vi "002_DataSave.vi"(11 "Queue Ref":T1={"UI"=refnum, "Message"=refnum, "Data"=refnum, "Caller"=refnum, "Name"="000 Common", "Data Path"=path "", "Class Path"=path "", "SubPanel"=refnum, "Project Name"="", "MNT"="", "Title"="", "Data Source"=refnum, "Queue List"={}, "VI"=refnum, "UE"=refnum}) -> ()   [LabVIEW 2020]
doc: "DataSave"
uses:
  Alin/QMH/000 Module Data Type.ctl
  Alin/QMH/Queue Message.ctl
  <vilib>/Utility/config.llb/Read Key (String).vi
  <vilib>/Utility/config.llb/Write Key (String).vi
  <vilib>/Utility/config.llb/NI_LVConfig.lvlib
panel:
  in  "Data Save Edit":bool
  in  "Open Save Folder":bool
  in  "Data Save List":i32(listbox)
  in  "Data Graph Edit":bool
  in  "Open Graph Folder":bool
  in  "Data Graph List":i32(listbox)
  in  "Data Save Launch":bool
  in  "Data Save Interval":sgl=100.0 caption="存储间隔" min=0.1 max=3600 step=0.1 format="%#_g s"
  in  "Data Save Refresh":bool
  in  "Panel Show":bool
  in  "Save Info":i32(listbox) caption="操作日志"
  in  "Data Save Log":i32(listbox)
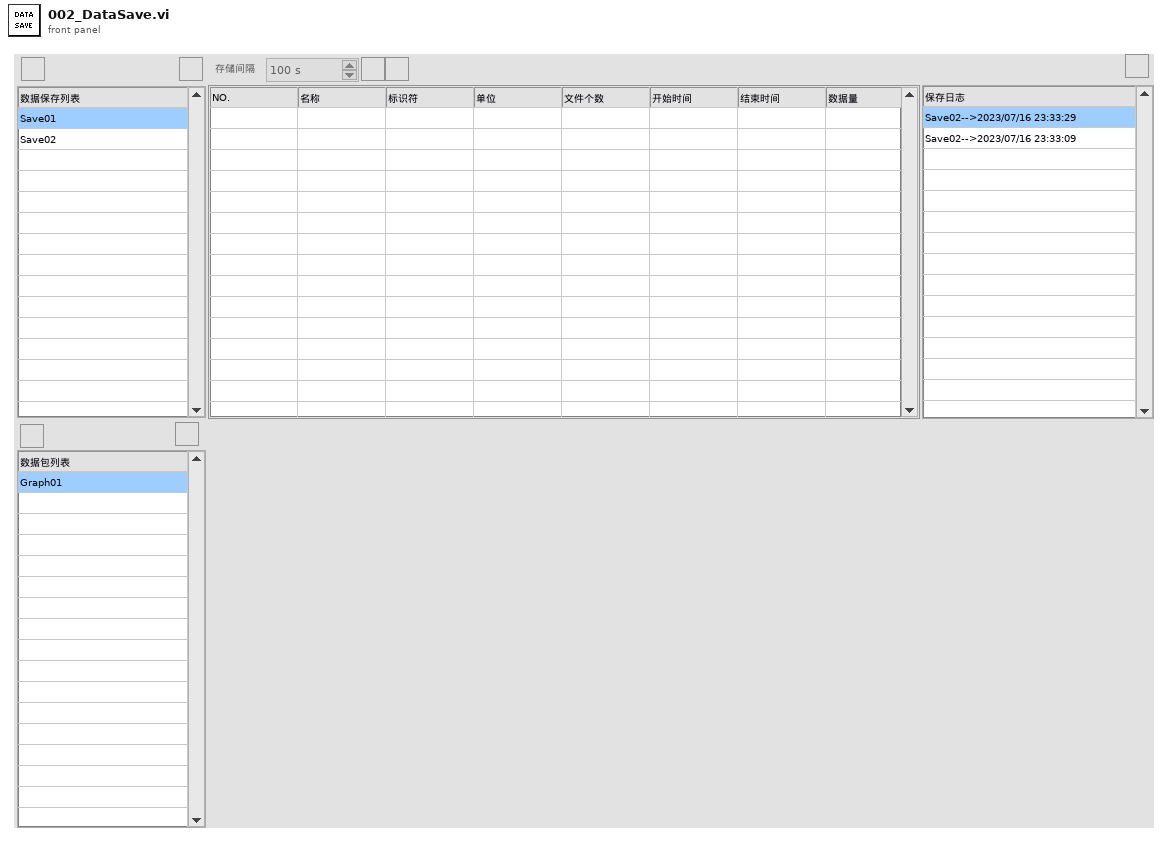
[diagram p1: front panel]
types:
  T1 = typedef "000 Module Data Type.ctl" = cluster{"UI":refnum<queue>, "Message":refnum<queue>, "Data":refnum<queue>, "Caller":refnum<queue>, "Name":string, "Data Path":path, "Class Path":path, "SubPanel":refnum<vi>, "Project Name":string, "MNT":string, "Title":string, "Data Source":refnum<queue>, "Queue List":map{string, refnum<queue>}, "VI":refnum<vi>, "UE":refnum<user-event>}
  T2 = cluster{"Queue":T1, "Data Save Log":refnum<vi>, "Log":string[]}
  T3 = typedef "eventvkey.ctl" = enum16{"ASCII", "Enter", "Return", "Shift", "Ctrl", "Alt", "Cmd", "Opt", "Caps", "NumLock", "Clear", "Break", "Up", "Down", "Left", "Right", "Insert", "Delete", "Home", "End", "PageUp", "PageDown", "Escape", "Help", "Pause", "ScrollLock", "F1", "F2", "F3", "F4", "F5", "F6", "F7", "F8", "F9", "F10", "F11", "F12", "F13", "F14", "F15", "F16", "F17", "F18", "F19", "F20", "F21", "F22", "F23", "F24", "Play", "VolumeUp", "VolumeDown", "Mute", "Two Byte Char"}
  T4 = cluster{"Shift":bool, "Ctrl":bool, "Alt":bool, "Cmd":bool, "Opt":bool}
  T5 = cluster{"Queue List":map{string, refnum<queue>}, "SubPanel":refnum<vi>, "Queue":T1, "Graph List":refnum<vi>, "Save List":refnum<vi>, "Save Info":refnum<vi>, "Active Save":string, "SQ":map{string, refnum<user-event>}}
  T6 = enum8{"Enabled", "Disabled", "Disabled and Grayed Out"}
  T7 = typedef "NI_LVConfig.lvlib/Config Data RefNum.ctl" = refnum<k1>
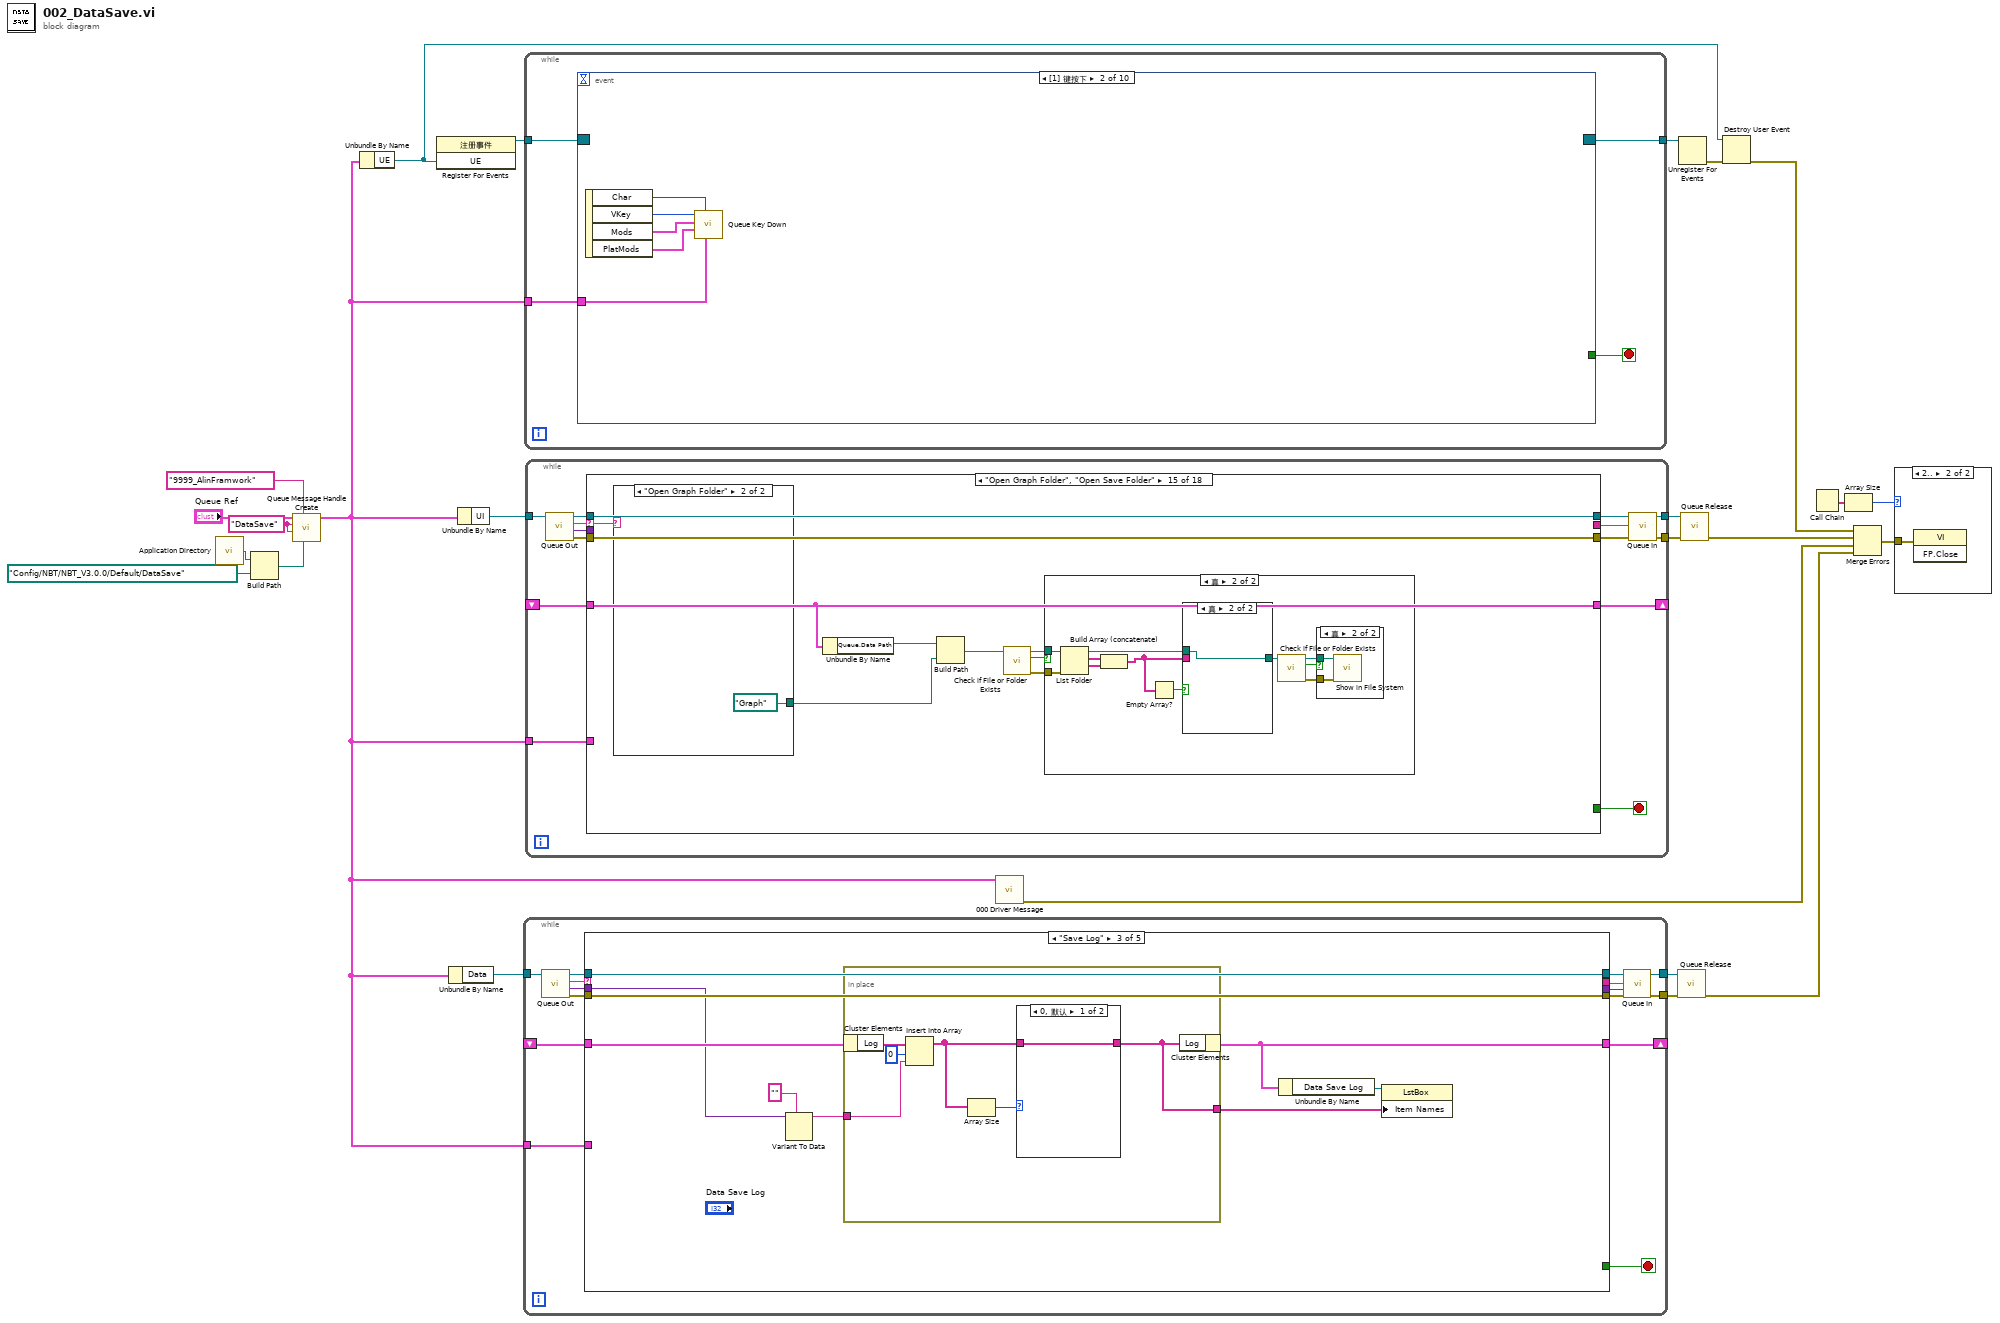
[diagram p0: block diagram]
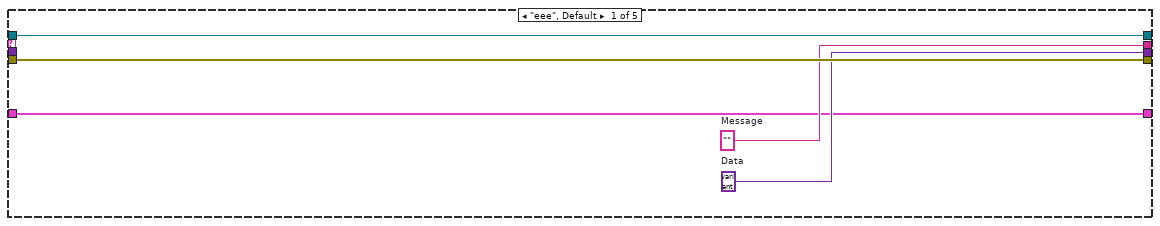
[diagram p2: hidden frame]
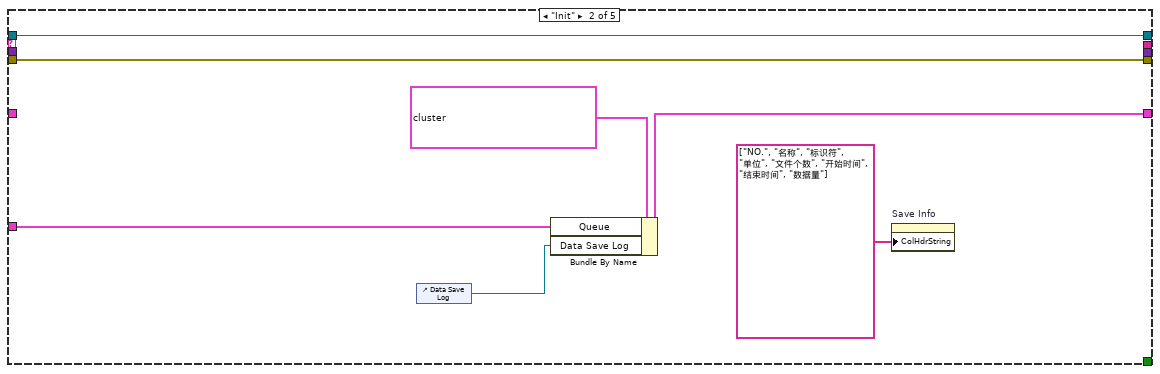
[diagram p3: hidden frame]
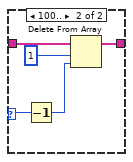
[diagram p4: hidden frame]
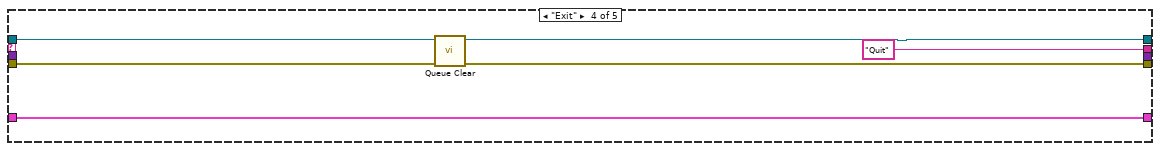
[diagram p5: hidden frame]
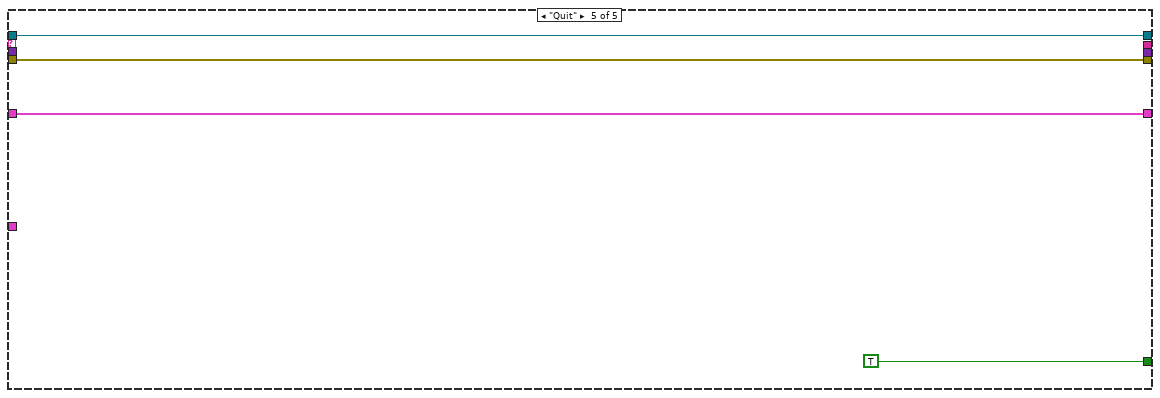
[diagram p6: hidden frame]
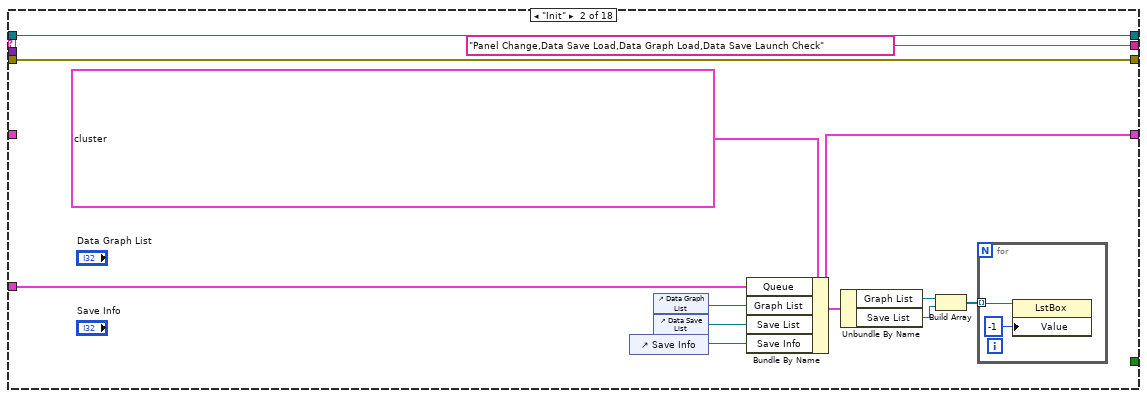
[diagram p9: hidden frame]
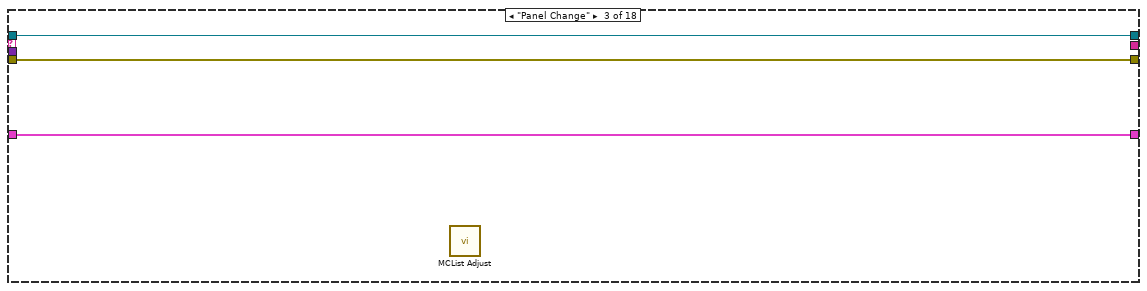
[diagram p10: hidden frame]
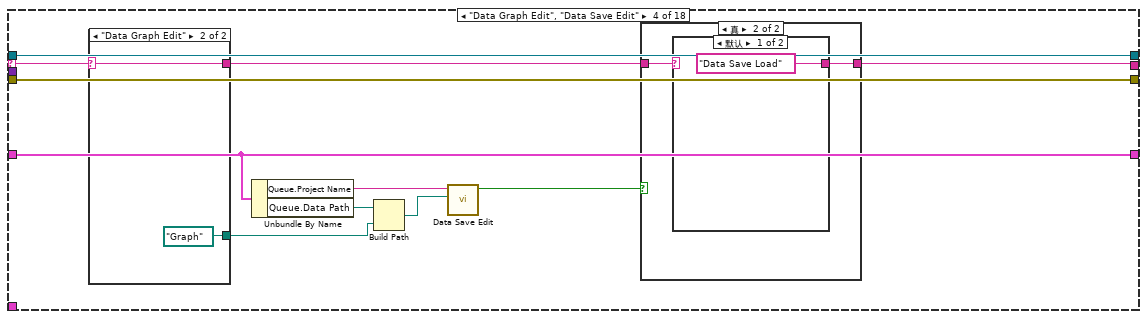
[diagram p11: hidden frame]
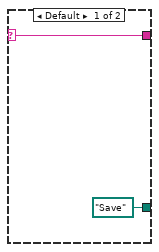
[diagram p12: hidden frame]
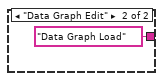
[diagram p14: hidden frame]
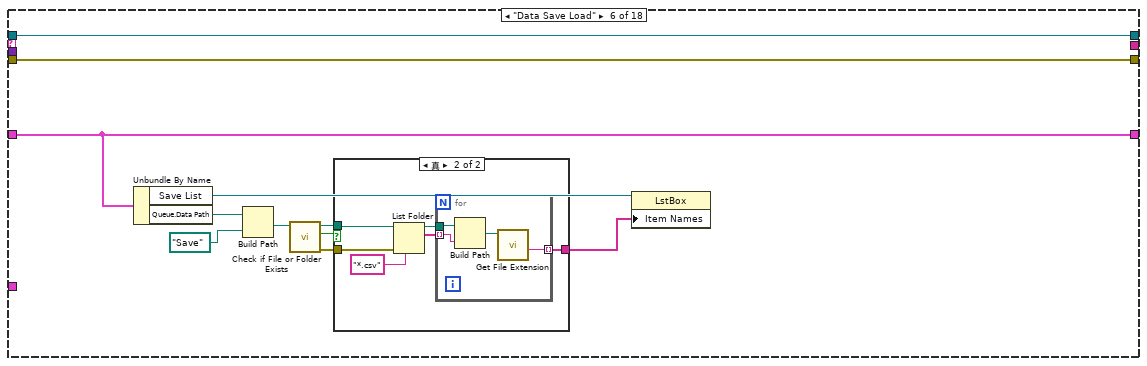
[diagram p16: hidden frame]
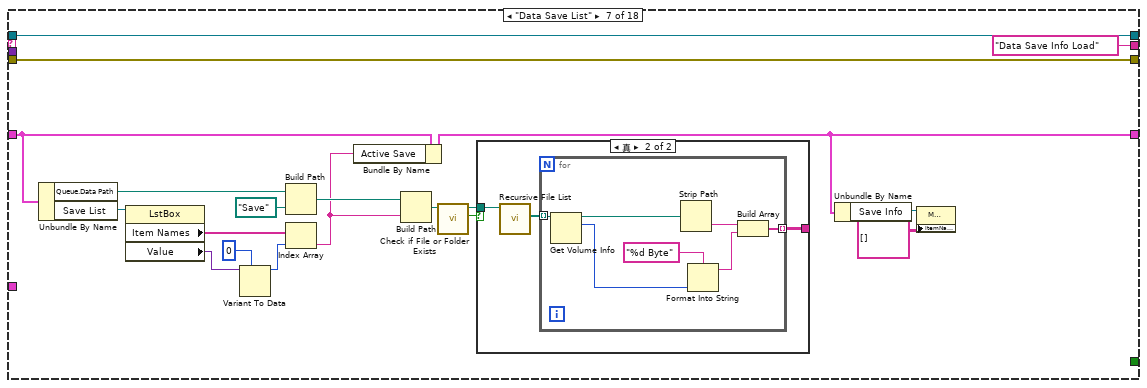
[diagram p18: hidden frame]
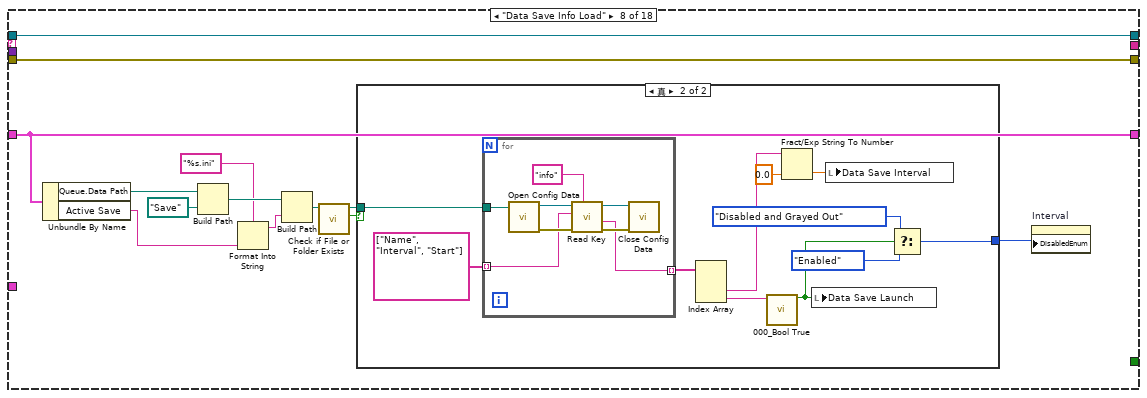
[diagram p20: hidden frame]
diagram:
  w2 = "DataSave" ("Title")
  n1 = call <vilib>:"Application Directory.vi"() -> ("Application Directory"=w5:path)
  n2 = Build Path(base path=w5, name or relative path=path "Config/NBT/NBT_V3.0.0/Default/DataSave" ("名称或相对路径")) -> (appended path=w3:path)
  n3 = call "Queue Message Handle Create.vi"("Data Path"=w3, "Project Name"="9999_AlinFramwork", "Name"=w2, "Title"=w2, "Queue Ref In"="Queue Ref") -> ("Queue Ref Out"=w7:T1)  [unwired: 5 in, 1 out]
  n4 = Unbundle By Name(w7) -> ("UE"=w6:refnum<user-event>)
  n5 = register-events(w6) -> (reference out=w9:refnum<event-registration>)  [unwired: 2 in, 1 out]
  n6 = Unbundle By Name(w7) -> ("Data"=w22:refnum<queue>)
  n7 = Unbundle By Name(w7) -> ("UI"=w14:refnum<queue>)
  n8 = while {
    tunnel: w22 -> [w35]
    tunnel: [w32] -> w20
    tunnel: [w31] -> w21
    shift-right: [w27] -> _
    shift-left: _ -> [w26]
    tunnel: w7 -> [w25]
    stop <- w39 stop-if-true
    n9 = call "Queue Out.vi"("Queue In"=w35) -> ("error out"=w38:errorcluster, "Data"=w36:variant, "Message"=w37:string, "Queue Out"=w34:refnum<queue>)  [unwired: 6 in, 1 out]
    n10 = case shown="\"Save Log\"" w37 {
      tunnel: w34 -> [w44 w51 w60 w77 w81]
      tunnel: w38 -> [w43 w50 w59 w75 w82]
      tunnel: [w44 w51 w60 w76 w81] -> w33
      tunnel: [w43 w50 w59 w74 w82] -> w30
      tunnel: [w42 _ _ "Quit" _] -> w29
      tunnel: [_ _ _ _ TRUE] -> w39
      tunnel: [w41 _ _ _ _] -> w28
      tunnel: w36 -> [_ _ w57 _ _]
      tunnel: [w40 w47 w54 w73 w79] -> w27
      tunnel: w26 -> [w40 _ w58 w73 w79]
      tunnel: w25 -> [_ w48 _ _ _]
      frame "eee", Default {
        w41 = variant  # Data
        w42 = ""  # Message
      }
      frame "Init" {
        n11 = control-ref of="Data Save Log"() -> (w45:refnum<vi>)
        n12 = Bundle By Name(cluster=T2 {"Queue"={"UI"=refnum, "Message"=refnum, "Data"=refnum, "Caller"=refnum, "Name"="", "Data Path"=path "", "Class Path"=path "", "SubPanel"=refnum, "Project Name"="", "MNT"="", "Title"="", "Data Source"=refnum, "Queue List"={}, "VI"=refnum, "UE"=refnum}, "Data Save Log"=refnum, "Log"=[]}, "Queue"=w48, "Data Save Log"=w45) -> (w47:T2)
        n13 = property on="Save Info" class="MCListbox (严格)"("ColHdrString"=string[] ["NO.", "名称", "标识符", "单位", "文件个数", "开始时间", "结束时间", "数据量"] ("列首字符串[]")) -> ()  [unwired: 2 in, 2 out]
      }
      frame "Save Log" {
        n14 = Variant To Data(type="", Variant=w57) -> (data=w55:string)  [unwired: 1 in, 1 out]
        n15 = in-place {
          in-place-border: w55 -> [w65]
          in-place-border: [w61] -> w52
          n16 = in-place-cluster #1(w58) -> ("Log"=w66:string[])
          n17 = Insert Into Array(array=w66, index=0 ("索引"), new element=w65) -> (w63:string[])
          n18 = Array Size(array=w63) -> (size(s)=w62:i32)
          n19 = case shown="0, 默认" w62 {
            selector: w62 -> [_ w69]
            tunnel: w63 -> [w67 w72]
            tunnel: [w67 w71] -> w61
            frame 0, Default {
            }
            frame 100.. {
              n20 = Decrement(x=w69) -> (x-1=w68:i32)
              n21 = Delete From Array(array=w72, length=1 ("长度"), index=w68) -> (array with subset deleted=w71:string[])  [unwired: 1 out]
            }
          }
          n22 = in-place-cluster #1("Log"=w61) -> (w54:T2)
        }
        n23 = Unbundle By Name(w54) -> ("Data Save Log"=w53:refnum<vi>)
        n24 = property class="LstBox"(reference=w53, "Item Names"=w52) -> ()  [unwired: 1 in, 2 out]
      }
      frame "Exit" {
        n25 = call "Queue Clear.vi"("error in (no error)"=w75, "Queue In"=w77) -> ("error out"=w74:errorcluster, "Queue Out"=w76:refnum<queue>)  [unwired: 8 in]
      }
      frame "Quit" {
      }
    }
    n26 = call "Queue In.vi"("error in (no error)"=w30, "Data"=w28, "Message"=w29, "Queue In"=w33) -> ("error out"=w31:errorcluster, "Queue Out"=w32:refnum<queue>)  [unwired: 6 in]
  }
  n27 = while {
    tunnel: w9 -> [w86]
    tunnel: [w84] -> w10
    tunnel: w7 -> [w83]
    stop <- w85 stop-if-true
    n28 = event shown="[1] 键按下" {
      selector: w86 -> [_ _ _ _ _ _ _ _ _ _]
      dyn-events: [_ _ _ _ _ _ _ _ _ _] -> w84
      timeout: _ -> [_ _ _ _ _ _ _ _ _ _]
      tunnel: [_ _ _ _ _ w103 _ _ _ _] -> w85
      tunnel: w83 -> [_ w90 w95 w99 w102 _ w107 w117 w120 w124]
      event Timeout {
        n29 = event-data() -> ()  [unwired: 1 in, 1 out]
      }
      event Key Down {
        n30 = event-data() -> ("Char"=w91:i16, "VKey"=w89:T3, "Mods"=w88:cluster{"Num Pad":bool, "Menu Key":bool}, "PlatMods"=w87:T4)  [unwired: 1 in]
        n31 = call "Queue Key Down.vi"("Queue Ref Out"=w90, "C"=w91, "Platform Key"=w87, "Group Key"=w88, "V Key"=w89) -> ()  [unwired: 6 in, 1 out]
      }
      event "Data Save Edit", "Data Graph Edit", "Data Save Launch", "Data Save Refresh": Value Change {
        n32 = event-data() -> ("CtlRef"=w94:refnum<vi>)  [unwired: 1 in]
        n33 = Unbundle By Name(w95) -> ("UI"=w93:refnum<queue>)
        n34 = property class="Bool"(reference=w94) -> ("Label.Text"=w92:string)  [unwired: 1 in, 2 out]
        n35 = call "Queue In.vi"("Message"=w92, "Queue In"=w93) -> ()  [unwired: 8 in, 2 out]
      }
      event "Data Save Interval": Value Change {
        n36 = event-data() -> ("CtlRef"=w97:refnum<vi>)  [unwired: 1 in]
        n37 = Unbundle By Name(w99) -> ("UI"=w98:refnum<queue>)
        n38 = property class="DigNum (严格)"(reference=w97) -> ("Label.Text"=w96:string)  [unwired: 1 in, 2 out]
        n39 = call "Queue In.vi"("Message"=w96, "Queue In"=w98) -> ()  [unwired: 8 in, 2 out]
      }
      event Panel Resize {
        n40 = event-data() -> ()  [unwired: 1 in, 1 out]
        n41 = Unbundle By Name(w102) -> ("Message"=w101:refnum<queue>)
        n42 = call "Queue In.vi"("Message"="Panel Change", "Queue In"=w101) -> ()  [unwired: 8 in, 2 out]
      }
      event User Event {
        n43 = event-data() -> ("Message"=w105:string)  [unwired: 1 in]
        n44 = Equal?(x=w105, y="Exit") -> (x = y?=w103:bool)
      }
      event Panel Close? {
        n45 = event-data() -> ()  [unwired: 1 in, 1 out]
        n46 = Unbundle By Name(w107) -> ("Message"=w106:refnum<queue>)
        n47 = Call Chain() -> (call chain=w110:string[])
        n48 = Array Size(array=w110) -> (size(s)=w109:i32)
        n49 = case shown="0, 默认" w109 {
          tunnel: ["Exit Prepare" ("Message") "Panel Hidden" ("Message")] -> w108
          frame 0, Default {
          }
          frame 2.. {
          }
        }
        n50 = call "Queue In.vi"("Message"=w108, "Queue In"=w106) -> ()  [unwired: 8 in, 2 out]
        n51 = event-data("Discard?"=TRUE ("放弃？")) -> ()  [unwired: 1 in, 1 out]
      }
      event "Data Save List", "Data Graph List", "Open Save Folder", "Open Graph Folder": Value Change {
        n52 = event-data() -> ("CtlRef"=w116:refnum<vi>)  [unwired: 1 in, 2 out]
        n53 = Unbundle By Name(w117) -> ("UI"=w115:refnum<queue>)
        n54 = property class="Ctl"(reference=w116) -> ("Label.Text"=w114:string)  [unwired: 1 in, 2 out]
        n55 = call "Queue In.vi"("Message"=w114, "Queue In"=w115) -> ()  [unwired: 8 in, 2 out]
      }
      event "Data Save List": Double Click {
        n56 = event-data() -> ()  [unwired: 1 in, 1 out]
        n57 = Unbundle By Name(w120) -> ("UI"=w119:refnum<queue>)
        n58 = call "Queue In.vi"("Message"="Show Panel", "Queue In"=w119) -> ()  [unwired: 8 in, 2 out]
      }
      event "Panel Show": Value Change {
        n59 = event-data() -> ("CtlRef"=w122:refnum<vi>)  [unwired: 1 in]
        n60 = Unbundle By Name(w124) -> ("Message"=w123:refnum<queue>)
        n61 = property class="Bool"(reference=w122) -> ("Label.Text"=w121:string)  [unwired: 1 in, 2 out]
        n62 = call "Queue In.vi"("Message"=w121, "Queue In"=w123) -> ()  [unwired: 8 in, 2 out]
      }
    }
  }
  n63 = while {
    tunnel: w14 -> [w134]
    tunnel: [w131] -> w12
    tunnel: [w130] -> w13
    tunnel: w7 -> [w127]
    shift-right: [w126] -> _
    shift-left: _ -> [w125]
    stop <- w138 stop-if-true
    n64 = call "Queue Out.vi"("Queue In"=w134) -> ("error out"=w137:errorcluster, "Data"=w135:variant, "Message"=w136:string, "Queue Out"=w133:refnum<queue>)  [unwired: 6 in, 1 out]
    n65 = case shown="\"Open Graph Folder\", \"Open Save Folder\"" w136 {
      selector: w136 -> [_ _ _ w161 _ _ _ _ _ _ _ _ _ w415 w425 _ w457 _]
      tunnel: w133 -> [w141 w153 w158 w169 w180 w191 w220 w243 w269 w282 w316 w343 w404 w421 w433 w456 w467 w477]
      tunnel: w137 -> [w140 w152 w157 w168 w179 w190 w219 w242 w268 w281 w315 w342 w403 w420 w432 w455 w465 w478]
      tunnel: [w141 w153 w158 w169 w180 w191 w220 w243 w269 w282 w316 w343 w404 w421 w433 w456 w466 w477] -> w132
      tunnel: [w140 w152 w157 w168 w179 w190 w219 w242 w268 w281 w315 w342 w403 w420 w432 w455 w464 w478] -> w129
      tunnel: [_ "Panel Change,Data Save Load,Data Graph Load,Data Save Launch Check" _ w162 _ _ "Data Save Info Load" _ w265 _ "Data Save Info Load,Data Save Launch Check" _ _ _ _ _ "Quit" _] -> w128
      tunnel: [_ _ _ _ _ _ _ _ _ _ _ _ _ _ _ _ _ TRUE] -> w138
      tunnel: w135 -> [_ _ _ _ _ _ _ _ _ _ _ _ _ _ _ _ _ _]
      tunnel: w127 -> [_ w150 _ _ _ _ _ _ _ _ _ _ _ _ _ _ _ _]
      tunnel: [w139 w145 w156 w167 w178 w189 w203 w237 w264 w279 w307 w340 w402 w419 w431 w454 w459 w475] -> w126
      tunnel: w125 -> [w139 _ w156 w167 w178 w189 w207 w237 w264 w280 w307 w331 w402 w419 w431 w454 w459 w475]
      frame "eee", Default {
      }
      frame "Init" {
        n66 = control-ref of="Save Info"() -> (w146:refnum<vi>)
        n67 = control-ref of="Data Graph List"() -> (w148:refnum<vi>)
        n68 = control-ref of="Data Save List"() -> (w147:refnum<vi>)
        n69 = Bundle By Name(cluster=T5 {"Queue List"={}, "SubPanel"=refnum, "Queue"={"UI"=refnum, "Message"=refnum, "Data"=refnum, "Caller"=refnum, "Name"="", "Data Path"=path "", "Class Path"=path "", "SubPanel"=refnum, "Project Name"="", "MNT"="", "Title"="", "Data Source"=refnum, "Queue List"={}, "VI"=refnum, "UE"=refnum}, "Graph List"=refnum, "Save List"=refnum, "Save Info"=refnum, "Active Save"="", "SQ"={}}, "Queue"=w150, "Graph List"=w148, "Save List"=w147, "Save Info"=w146) -> (w145:T5)
        n70 = Unbundle By Name(w145) -> ("Graph List"=w144:refnum<vi>, "Save List"=w143:refnum<vi>)
        n71 = Build Array(w144, w143) -> (w142:refnum<vi>[])
        n72 = for {
          tunnel: w142 -> [w155] mode=indexing
          n73 = property class="LstBox"(reference=w155, "Value"=-1) -> ()  [unwired: 1 in, 2 out]
        }
      }
      frame "Panel Change" {
        n74 = call "MCList Adjust.vi"() -> ()  [unwired: 11 in, 1 out]
      }
      frame "Data Graph Edit", "Data Save Edit" {
        n75 = case shown="\"Data Graph Edit\"" w161 {
          selector: w161 -> [w170 w172]
          tunnel: [path "Save" ("名称或相对路径") path "Graph" ("名称或相对路径")] -> w160
          tunnel: [w170 w172] -> w159
          frame Default {
          }
          frame "Data Graph Edit" {
          }
        }
        n76 = Unbundle By Name(w167) -> ("Queue.Project Name"=w166:string, "Queue.Data Path"=w164:path)
        n77 = Build Path(base path=w164, name or relative path=w160) -> (appended path=w163:path)
        n78 = call "Data Save Edit.vi"("Data Path"=w163, "Project"=w166) -> ("OK?"=w165:bool)  [unwired: 9 in]
        n79 = case shown="真" w165 {
          tunnel: [_ w175] -> w162
          tunnel: w159 -> [_ w174]
          frame False {
          }
          frame True {
            n80 = case shown="默认" w174 {
              tunnel: ["Data Save Load" "Data Graph Load"] -> w175
              frame Default {
              }
              frame "Data Graph Edit" {
              }
            }
          }
        }
      }
      frame "Data Save Delete" {
      }
      frame "Data Save Load" {
        n81 = Unbundle By Name(w189) -> ("Save List"=w182:refnum<vi>, "Queue.Data Path"=w188:path)
        n82 = Build Path(base path=w188, name or relative path=path "Save" ("名称或相对路径")) -> (appended path=w186:path)
        n83 = call <vilib>:"Check if File or Folder Exists.vi"("path"=w186) -> ("error out"=w183:errorcluster, "file or folder exists?"=w185:bool, "dup path"=w184:path)  [unwired: 8 in]
        n84 = case shown="真" w185 {
          tunnel: w184 -> [_ w197]
          tunnel: w183 -> [_ w196]
          tunnel: [_ w193] -> w181
          frame False {
          }
          frame True {
            n85 = List Folder(path=w197, pattern="*.csv" ("类型"), error in=w196) -> (path out=w194:path, filenames=w195:string[])  [unwired: 1 in, 2 out]
            n86 = for {
              tunnel: w195 -> [w200] mode=indexing
              tunnel: w194 -> [w201]
              tunnel: [w198] -> w193 mode=indexing
              n87 = Build Path(base path=w201, name or relative path=w200) -> (appended path=w199:path)
              n88 = call <vilib>:"Get File Extension.vi"("file"=w199) -> ("filename without extension"=w198:string)  [unwired: 6 in, 4 out]
            }
          }
        }
        n89 = property class="LstBox"(reference=w182, "Item Names"=w181) -> ()  [unwired: 1 in, 2 out]
      }
      frame "Data Save List" {
        n90 = Unbundle By Name(w207) -> ("Queue.Data Path"=w213:path, "Save List"=w218:refnum<vi>)
        n91 = property class="LstBox"(reference=w218) -> ("Item Names"=w217:string[], "Value"=w216:variant)  [unwired: 1 in, 2 out]
        n92 = Variant To Data(type=0 ("Data Save List"), Variant=w216) -> (data=w214:i32)  [unwired: 1 in, 1 out]
        n93 = Build Path(base path=w213, name or relative path=path "Save" ("名称或相对路径")) -> (appended path=w211:path)
        n94 = Index Array(array=w217, index=w214) -> (element=w202:string)
        n95 = Bundle By Name(cluster=w207, "Active Save"=w202) -> (w203:T5)
        n96 = Build Path(base path=w211, name or relative path=w202) -> (appended path=w210:path)
        n97 = call <vilib>:"Check if File or Folder Exists.vi"("path"=w210) -> ("file or folder exists?"=w209:bool, "dup path"=w208:path)  [unwired: 8 in, 1 out]
        n98 = case shown="真" w209 {
          tunnel: w208 -> [_ w223]
          tunnel: [_ w221] -> _
          frame False {
          }
          frame True {
            n99 = call <vilib>:"Recursive File List.vi"("Folder Path"=w223) -> ("All Files in Dir"=w222:path[])  [unwired: 6 in, 4 out]
            n100 = for {
              tunnel: w222 -> [w230] mode=indexing
              tunnel: [w224] -> w221 mode=indexing
              n101 = Get Volume Info(11:w230) -> (2:w227:i64, 3:w229:path)  [unwired: 1 in, 4 out]
              n102 = Strip Path(path=w229) -> (name=w226:string)  [unwired: 1 out]
              n103 = Format Into String(format string="%d Byte" ("格式字符串"), w227) -> (resulting string=w225:string)  [unwired: 2 in, 1 out]
              n104 = Build Array(w226, w225) -> (w224:string[])
            }
          }
        }
        n105 = Unbundle By Name(w203) -> ("Save Info"=w206:refnum<vi>)
        n106 = property class="MCListbox"(reference=w206, "ItemNames"=string[][] [] ("项名")) -> ()  [unwired: 1 in, 2 out]
      }
      frame "Data Save Info Load" {
        n107 = Unbundle By Name(w237) -> ("Queue.Data Path"=w241:path, "Active Save"=w232:string)
        n108 = Build Path(base path=w241, name or relative path=path "Save" ("名称或相对路径")) -> (appended path=w239:path)
        n109 = Format Into String(format string="%s.ini" ("格式字符串"), w232) -> (resulting string=w235:string)  [unwired: 2 in, 1 out]
        n110 = Build Path(base path=w239, name or relative path=w235) -> (appended path=w238:path)
        n111 = call <vilib>:"Check if File or Folder Exists.vi"("path"=w238) -> ("file or folder exists?"=w233:bool, "dup path"=w234:path)  [unwired: 8 in, 1 out]
        n112 = case shown="真" w233 {
          tunnel: w234 -> [_ w255]
          tunnel: [T6."Enabled" ("禁用") w245] -> w231
          frame False {
          }
          frame True {
            n113 = for {
              tunnel: w255 -> [w263]
              tunnel: string[] ["Name", "Interval", "Start"] -> [w257] mode=indexing
              tunnel: [w256] -> w253 mode=indexing
              n114 = call <vilib>:"Open Config Data.vi"("configuration file path"=w263) -> ("error out"=w261:errorcluster, "refnum"=w262:T7)  [unwired: 8 in, 1 out]
              n115 = call-poly <vilib>:"Read Key.vi"("section"="info", "error in (no error)"=w261, "key"=w257, "refnum"=w262) -> ("error out"=w260:errorcluster, "value"=w256:string, "refnum out"=w259:T7)  [unwired: 4 in, 1 out]
              n116 = call <vilib>:"Close Config Data.vi"("error in (no error)"=w260, "refnum"=w259) -> ()  [unwired: 8 in, 2 out]
            }
            n117 = Index Array(array=w253) -> (element #2=w252:string, element #3=w251:string)  [unwired: 3 in, 1 out]
            n118 = call "000_Bool True.vi"("Bool String"=w251) -> ("True"=w248:bool)  [unwired: 8 in, 2 out]
            n119 = Fract/Exp String To Number(string=w252, default (0 dbl)=sgl 0.0 ("偏移量")) -> (number=w250:sgl)  [unwired: 2 in, 1 out]
            n120 = local write "Data Save Launch"(w248) -> ()
            n121 = local write "Data Save Interval"(w250) -> ()
            n122 = Select(t=T6."Disabled and Grayed Out" ("禁用"), s=w248, f=T6."Enabled" ("禁用")) -> (s? t:f=w245:T6)
          }
        }
        n123 = property on="Interval" class="DigNum (严格)"("DisabledEnum"=w231) -> ()  [unwired: 2 in, 2 out]
      }
      frame "Data Save Launch" {
        n124 = local read "Data Save Launch"() -> (w267:bool)
        n125 = case shown="真" w267 {
          tunnel: [_ w277] -> w266
          tunnel: w264 -> [_ w276]
          frame False {
          }
          frame True {
            n126 = local read "Data Save Interval"() -> (w273:sgl)
            n127 = Unbundle By Name(w276) -> ("Active Save"=w274:string)
            n128 = Format Into String(format string="保存名称：%s\n保存间隔：%#.3f s" ("格式字符串"), w274, w273) -> (resulting string=w272:string)  [unwired: 2 in, 1 out]
            n129 = Two Button Dialog(message=w272) -> (T button?=w277:bool)  [unwired: 2 in]
          }
        }
        n130 = case shown="真" w266 {
          tunnel: ["Data Save Interval,Data Save Stop" "Data Save Interval"] -> w265
          frame False {
          }
          frame True {
          }
        }
        n131 = local write "Data Save Launch"(w266) -> ()
      }
      frame "Data Save Stop" {
        n132 = Unbundle By Name(w280) -> ("Active Save"=w278:string)
        n133 = in-place {
          in-place-border: w278 -> [w286]
          n134 = in-place-cluster #2(w280) -> ("SQ"=w287:map{string, refnum<user-event>})
          n135 = Remove From Map(10:w286, 11:w287) -> (1:w285:refnum<user-event>, 2:w283:bool, 3:w284:map{string, refnum<user-event>})
          n136 = case shown="假" w283 {
            tunnel: w285 -> [w289 _]
            frame False {
              n137 = Generate User Event(user event=w289, event data cluster="Exit" ("事件数据")) -> ()  [unwired: 2 in, 2 out]
            }
            frame True {
            }
          }
          n138 = in-place-cluster #2("SQ"=w284) -> (w279:T5)
        }
      }
      frame "Data Save Interval" {
        n139 = Unbundle By Name(w307) -> ("Queue.Data Path"=w309:path, "Save List"=w314:refnum<vi>)
        n140 = property class="LstBox"(reference=w314) -> ("Item Names"=w313:string[], "Value"=w312:variant)  [unwired: 1 in, 2 out]
        n141 = Variant To Data(type=0 ("Data Save List"), Variant=w312) -> (data=w310:i32)  [unwired: 1 in, 1 out]
        n142 = Build Path(base path=w309, name or relative path=path "Save" ("名称或相对路径")) -> (appended path=w301:path)
        n143 = Index Array(array=w313, index=w310) -> (element=w293:string)
        n144 = call <vilib>:"Check if File or Folder Exists.vi"("path"=w301) -> ("error out"=w298:errorcluster, "file or folder exists?"=w300:bool, "dup path"=w299:path)  [unwired: 8 in]
        n145 = case shown="假" w300 {
          tunnel: w299 -> [w320 w322]
          tunnel: w298 -> [w319 w321]
          tunnel: [w318 w322] -> w297
          tunnel: [w317 w321] -> _
          frame False {
            n146 = Create Folder(path (use dialog)=w320, error in=w319) -> (created path=w318:path, error out=w317:errorcluster)  [unwired: 1 in, 1 out]
          }
          frame True {
          }
        }
        n147 = call "000_Bool True.vi"("Value"="Data Save Launch") -> ("String Out"=w291:string)  [unwired: 8 in, 2 out]
        n148 = Format Into String(format string="%#.3f" ("格式字符串"), "Data Save Interval") -> (resulting string=w292:string)  [unwired: 2 in, 1 out]
        n149 = Format Into String(format string="%s.ini" ("格式字符串"), w293) -> (resulting string=w305:string)  [unwired: 2 in, 1 out]
        n150 = Build Array(w293, w292, w291) -> (w290:string[])
        n151 = Build Path(base path=w297, name or relative path=w305) -> (appended path=w302:path)
        n152 = for {
          tunnel: w302 -> [w330]
          tunnel: string[] ["Name", "Interval", "Start"] -> [w324] mode=indexing
          tunnel: w290 -> [w323] mode=indexing
          n153 = call <vilib>:"Open Config Data.vi"("configuration file path"=w330) -> ("error out"=w328:errorcluster, "refnum"=w329:T7)  [unwired: 8 in, 1 out]
          n154 = call-poly <vilib>:"Write Key.vi"("section"="info", "error in (no error)"=w328, "value"=w323, "key"=w324, "refnum"=w329) -> ("error out"=w327:errorcluster, "refnum out"=w326:T7)  [unwired: 4 in, 1 out]
          n155 = call <vilib>:"Close Config Data.vi"("error in (no error)"=w327, "refnum"=w326) -> ()  [unwired: 8 in, 2 out]
        }
      }
      frame "Data Save Launch Check" {
        n156 = Unbundle By Name(w331) -> ("Queue.Data Path"=w334:path)
        n157 = Build Path(base path=w334, name or relative path=path "Save" ("名称或相对路径")) -> (appended path=w333:path)
        n158 = call <vilib>:"Check if File or Folder Exists.vi"("path"=w333) -> ("error out"=w337:errorcluster, "file or folder exists?"=w335:bool, "dup path"=w336:path)  [unwired: 8 in]
        n159 = case shown="真" w335 {
          tunnel: "*.ini" ("类型") -> [_ w350]
          tunnel: [_ w349] -> w339
          tunnel: [w344 w348] -> w338
          tunnel: w337 -> [_ w346]
          tunnel: w336 -> [w344 w347]
          tunnel: [_ w345] -> _
          frame False {
          }
          frame True {
            n160 = List Folder(path=w347, pattern=w350, error in=w346) -> (path out=w348:path, filenames=w349:string[], error out=w345:errorcluster)  [unwired: 1 in, 1 out]
          }
        }
        n161 = for {
          shift-right: [w355] -> w340
          shift-left: w331 -> [w356]
          tunnel: w339 -> [w366] mode=indexing
          tunnel: w338 -> [w352]
          tunnel: w331 -> [w351]
          n162 = Build Path(base path=w352, name or relative path=w366) -> (appended path=w359:path)
          n163 = call <vilib>:"Get File Extension.vi"("file"=w359) -> ("filename without extension"=w354:string)  [unwired: 6 in, 4 out]
          n164 = call <vilib>:"Open Config Data.vi"("configuration file path"=w359) -> ("error out"=w364:errorcluster, "refnum"=w365:T7)  [unwired: 8 in, 1 out]
          n165 = call-poly <vilib>:"Read Key.vi"("section"="info", "error in (no error)"=w364, "key"="Start", "refnum"=w365) -> ("error out"=w363:errorcluster, "value"=w358:string, "refnum out"=w362:T7)  [unwired: 4 in, 1 out]
          n166 = Build Path(base path=w352, name or relative path=w354) -> (appended path=w353:path)
          n167 = call <vilib>:"Close Config Data.vi"("error in (no error)"=w363, "refnum"=w362) -> ()  [unwired: 8 in, 2 out]
          n168 = call "000_Bool True.vi"("Bool String"=w358) -> ("True"=w357:bool)  [unwired: 8 in, 2 out]
          n169 = case shown="真" w357 {
            tunnel: w356 -> [w367 w372]
            tunnel: [w367 w371] -> w355
            tunnel: w354 -> [_ w370]
            tunnel: w353 -> [_ w369]
            tunnel: w351 -> [_ w368]
            frame False {
            }
            frame True {
              n170 = in-place {
                in-place-border: w370 -> [w375]
                in-place-border: w369 -> [w374]
                in-place-border: w368 -> [w373]
                n171 = in-place-cluster #3(w372) -> ("SQ"=w378:map{string, refnum<user-event>})
                n172 = Look In Map(map=w378, key=w375) -> (key not found?=w376:bool)  [unwired: 1 in, 1 out]
                n173 = case shown="真" w376 {
                  tunnel: w378 -> [w379 w393]
                  tunnel: [w379 w392] -> w377
                  tunnel: w375 -> [_ w385]
                  tunnel: w374 -> [_ w383]
                  tunnel: w373 -> [_ w382]
                  frame False {
                  }
                  frame True {
                    w386 = ""  # Exit
                    n174 = vi-ref "002 DataSaveThread.vi"() -> (w389:refnum<vi>)
                    n175 = property class="VI"(reference=w389) -> ("Path"=w391:path)  [unwired: 1 in, 2 out]
                    n176 = Unbundle By Name(w382) -> ("Queue.Project Name"=w381:string, "Queue.Data"=w380:refnum<queue>)
                    n177 = Create User Event(user event datatype=w386) -> (user event=w384:refnum<user-event>)  [unwired: 1 in, 1 out]
                    n178 = Open VI Reference(type specifier VI Refnum (for type only)=refnum<vi> refnum ("类型说明符VI引用句柄（仅用于类型）"), vi path=w391, options=128 ("选项")) -> (vi reference=w390:refnum<vi>)  [unwired: 3 in, 1 out]
                    n179 = Insert Into Map(map in=w393, key=w385, value=w384) -> (map out=w392:map{string, refnum<user-event>})  [unwired: 2 out]
                    n180 = call-by-ref "开始异步调用"(reference=w390, "Caller"=w380, "Project"=w381, "Path"=w383, "Exit"=w384) -> ()  [unwired: 9 in, 2 out]
                  }
                }
                n181 = in-place-cluster #3("SQ"=w377) -> (w371:T5)
              }
            }
          }
        }
      }
      frame "Data Graph Load" {
        n182 = Unbundle By Name(w402) -> ("Graph List"=w395:refnum<vi>, "Queue.Data Path"=w401:path)
        n183 = Build Path(base path=w401, name or relative path=path "Graph" ("名称或相对路径")) -> (appended path=w399:path)
        n184 = call <vilib>:"Check if File or Folder Exists.vi"("path"=w399) -> ("error out"=w396:errorcluster, "file or folder exists?"=w398:bool, "dup path"=w397:path)  [unwired: 8 in]
        n185 = case shown="真" w398 {
          tunnel: w397 -> [_ w409]
          tunnel: w396 -> [_ w408]
          tunnel: [_ w405] -> w394
          frame False {
          }
          frame True {
            n186 = List Folder(path=w409, error in=w408) -> (path out=w406:path, filenames=w407:string[])  [unwired: 2 in, 2 out]
            n187 = for {
              tunnel: w407 -> [w412] mode=indexing
              tunnel: w406 -> [w413]
              tunnel: [w410] -> w405 mode=indexing
              n188 = Build Path(base path=w413, name or relative path=w412) -> (appended path=w411:path)
              n189 = call <vilib>:"Get File Extension.vi"("file"=w411) -> ("filename without extension"=w410:string)  [unwired: 6 in, 4 out]
            }
          }
        }
        n190 = property class="LstBox"(reference=w395, "Item Names"=w394) -> ()  [unwired: 1 in, 2 out]
      }
      frame "Show Panel" {
        n191 = Unbundle By Name(w419) -> ("SQ"=w418:map{string, refnum<user-event>}, "Active Save"=w417:string)
        n192 = Look In Map(map=w418, key=w417) -> (key not found?=w414:bool, value=w416:refnum<user-event>)  [unwired: 1 in]
        n193 = case shown="假" w414 {
          tunnel: w416 -> [w423 _]
          tunnel: w415 -> [w422 _]
          frame False {
            n194 = Generate User Event(user event=w423, event data cluster=w422) -> ()  [unwired: 2 in, 2 out]
          }
          frame True {
          }
        }
      }
      frame "Open Graph Folder", "Open Save Folder" {
        n195 = case shown="\"Open Graph Folder\"" w425 {
          tunnel: [path "Save" ("名称或相对路径") path "Graph" ("名称或相对路径")] -> w424
          frame Default {
          }
          frame "Open Graph Folder" {
          }
        }
        n196 = Unbundle By Name(w431) -> ("Queue.Data Path"=w427:path)
        n197 = Build Path(base path=w427, name or relative path=w424) -> (appended path=w426:path)
        n198 = call <vilib>:"Check if File or Folder Exists.vi"("path"=w426) -> ("error out"=w428:errorcluster, "file or folder exists?"=w429:bool, "dup path"=w430:path)  [unwired: 8 in]
        n199 = case shown="真" w429 {
          tunnel: w430 -> [_ w446]
          tunnel: w428 -> [_ w445]
          frame False {
          }
          frame True {
            n200 = List Folder(path=w446, error in=w445) -> (path out=w444:path, filenames=w439:string[], folder names=w438:string[])  [unwired: 2 in, 1 out]
            n201 = Build Array (concatenate)(w439, w438) -> (w437:string[])
            n202 = Empty Array?(array=w437) -> (empty?=w436:bool)
            n203 = case shown="真" w436 {
              tunnel: w444 -> [w450 w451]
              tunnel: [w448 w451] -> w443
              tunnel: w437 -> [w447 _]
              frame False {
                n204 = Index Array(array=w447) -> (element=w449:string)  [unwired: 1 in]
                n205 = Build Path(base path=w450, name or relative path=w449) -> (appended path=w448:path)
              }
              frame True {
              }
            }
            n206 = call <vilib>:"Check if File or Folder Exists.vi"("path"=w443) -> ("error out"=w441:errorcluster, "file or folder exists?"=w440:bool, "dup path"=w442:path)  [unwired: 8 in]
            n207 = case shown="真" w440 {
              tunnel: w442 -> [_ w453]
              tunnel: w441 -> [_ w452]
              frame False {
              }
              frame True {
                n208 = call <vilib>:"Show in File System.vi"("error in (no error)"=w452, "file or directory path"=w453) -> ()  [unwired: 9 in, 1 out]
              }
            }
          }
        }
      }
      frame "====System====" {
      }
      frame "Exit" {
        n209 = Unbundle By Name(w459) -> ("Queue.UE"=w460:refnum<user-event>, "Queue.Message"=w463:refnum<queue>, "Queue.Data"=w462:refnum<queue>)
        n210 = Build Array(w463, w462) -> (w461:refnum<queue>[])
        n211 = Generate User Event(user event=w460, event data cluster=w457) -> ()  [unwired: 2 in, 2 out]
        n212 = for {
          tunnel: w461 -> [w474] mode=indexing
          tunnel: w457 -> [w473]
          n213 = call "Queue In.vi"("First"=TRUE, "Message"=w473, "Queue In"=w474) -> ()  [unwired: 7 in, 2 out]
        }
        n214 = Unbundle By Name(w459) -> ("SQ"=w458:map{string, refnum<user-event>})
        n215 = call "Queue Clear.vi"("error in (no error)"=w465, "Queue In"=w467) -> ("error out"=w464:errorcluster, "Queue Out"=w466:refnum<queue>)  [unwired: 8 in]
        n216 = for {
          tunnel: w458 -> [w471] mode=indexing
          tunnel: w457 -> [w469]
          n217 = Unbundle By Name(w471) -> ("UE"=w470:refnum<user-event>)
          n218 = Generate User Event(user event=w470, event data cluster=w469) -> ()  [unwired: 2 in, 2 out]
        }
      }
      frame "Quit" {
      }
    }
    n219 = call "Queue In.vi"("error in (no error)"=w129, "Message"=w128, "Queue In"=w132) -> ("error out"=w130:errorcluster, "Queue Out"=w131:refnum<queue>)  [unwired: 7 in]
  }
  n220 = call "000 Driver Message.vi"("Queue In"=w7) -> ("error out"=w23:errorcluster)  [unwired: 8 in, 2 out]
  n221 = call "Queue Release.vi"("error in (no error)"=w21, "Queue In"=w20) -> ("error out"=w24:errorcluster)  [unwired: 9 in]
  n222 = Unregister For Events(event registration refnum=w10) -> (error out=w11:errorcluster)  [unwired: 1 in]
  n223 = call "Queue Release.vi"("error in (no error)"=w13, "Queue In"=w12) -> ("error out"=w16:errorcluster)  [unwired: 9 in]
  n224 = Destroy User Event(user event=w6, error in=w11) -> (error out=w15:errorcluster)
  n225 = Call Chain() -> (call chain=w18:string[])
  n226 = Array Size(array=w18) -> (size(s)=w19:i32)
  n227 = Merge Errors(w15, w16, w23, w24) -> (w17:errorcluster)
  n228 = case shown="2.." w19 {
    tunnel: w17 -> [_ w479]
    frame 0, Default {
    }
    frame 2.. {
      n229 = invoke class="VI" method="FP.Close"(error in=w479) -> ()  [unwired: 2 in, 3 out]
    }
  }
